vi "conditional_struct.vi"() -> ()   [LabVIEW 2025]
panel:
  in  "dial":dbl(knob) min=0.0 max=10.0 step=1.0 scale=0.0..10.0
  out "led":bool
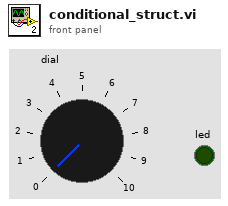
[diagram p1: front panel]
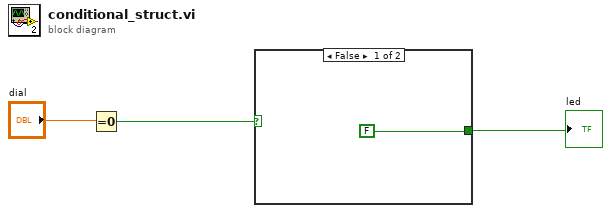
[diagram p0: block diagram]
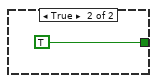
[diagram p2: hidden frame]
diagram:
  n1 = Equal To 0?(x="dial") -> (x = 0?=w2:bool)
  n2 = case shown="False" w2 {
    tunnel: [FALSE TRUE] -> w1
    frame False {
    }
    frame True {
    }
  }
  "led" <- w1
